vi "Check Confluence Settings.vi"(7 "Settings Path":path, 8 "Error in":errorcluster caption="Error in (no error)", 11 "Confluence Settings":T1) -> (0 "Error out":errorcluster, 3 "String":string)   [LabVIEW 2023]
uses:
  Confluence Settings.ctl
  <userlib>/_PetranWay/LabVIEW Confluence API/Source/Confluence/Confluence Connection/Confluence.lvclass
  <vilib>/DMC/VIDoc/Printers/Confluence/Confluence Printer Settings/VIDoc Settings - Confluence.lvclass
  <vilib>/DMC/VIDoc/Printers/Confluence/Confluence Printer/VIDoc Printer - Confluence.lvclass
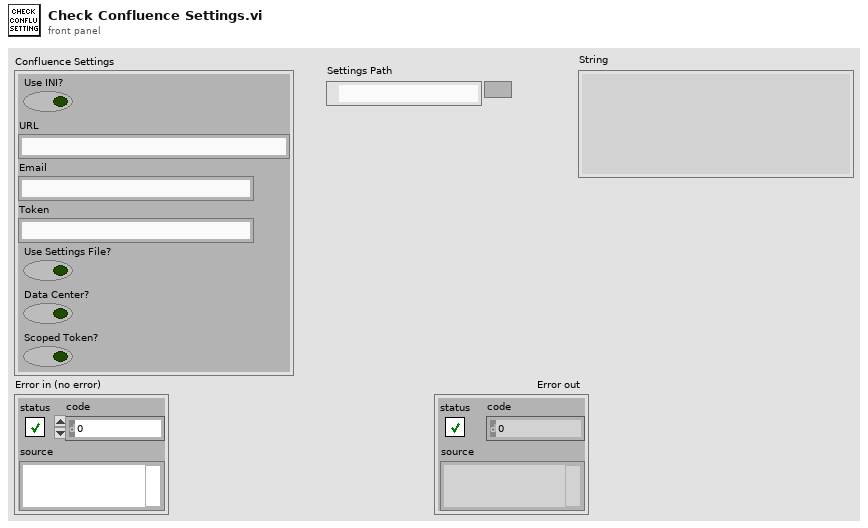
[diagram p1: front panel]
types:
  T1 = typedef "Confluence Settings.ctl" = cluster{"Use INI?":bool, "URL":string, "Email":string, "Token":string, "Use Settings File?":bool, "Data Center?":bool, "Scoped Token?":bool}
  T2 = typedef "VIDoc Printer - Confluence.lvlib/VIDoc Settings - Confluence.lvclass/Confluence Connection Settings.ctl" = cluster{"Connection Type":enum16{"Data Center", "Cloud"}, "URL":string, "Email":string}
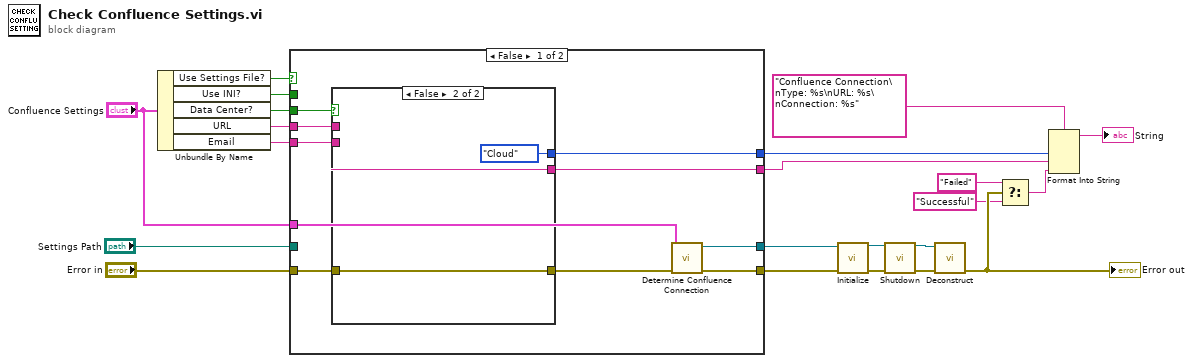
[diagram p0: block diagram]
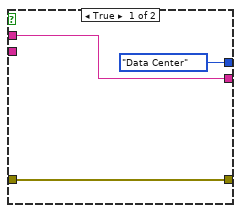
[diagram p2: hidden frame]
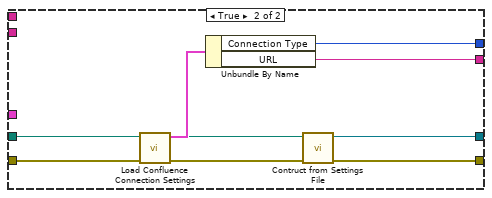
[diagram p3: hidden frame]
diagram:
  n1 = Unbundle By Name("Confluence Settings") -> ("Use Settings File?"=w22:bool, "Use INI?"=w21:bool, "Data Center?"=w20:bool, "URL"=w19:string, "Email"=w18:string)
  n2 = case shown="False" w22 {
    tunnel: [w25 w40] -> w3
    tunnel: "Error in" -> [w29 w44]
    tunnel: w21 -> [_ _]
    tunnel: w20 -> [w32 _]
    tunnel: w19 -> [w31 _]
    tunnel: w18 -> [w30 _]
    tunnel: "Settings Path" -> [_ w42]
    tunnel: [w28 w46] -> w14
    tunnel: [w27 w45] -> w13
    tunnel: [w24 w39] -> w2
    tunnel: "Confluence Settings" -> [w23 _]
    frame False {
      n3 = case shown="False" w32 {
        tunnel: w31 -> [w33 w36]
        tunnel: w30 -> [_ _]
        tunnel: w29 -> [w34 w38]
        tunnel: [w34 w38] -> w26
        tunnel: [enum16{"Data Center", "Cloud"}."Data Center" ("Connection Type") enum16{"Data Center", "Cloud"}."Cloud" ("Connection Type")] -> w28
        tunnel: [w33 w36] -> w27
        frame True {
        }
        frame False {
        }
      }
      n4 = call "Determine Confluence Connection.vi"("Error in"=w26, "Confluence Settings"=w23) -> ("Error out"=w25:errorcluster, "Confluence"=w24:refnum<class "Confluence.lvclass">)  [unwired: 8 in]
    }
    frame True {
      n5 = call <vilib>:"Load Confluence Connection Settings.vi"("Error in"=w44, "Settings Path"=w42) -> ("Error out"=w41:errorcluster, "Confluence Connection Settings"=w43:T2)  [unwired: 7 in, 1 out]
      n6 = Unbundle By Name(w43) -> ("Connection Type"=w46:enum16{"Data Center", "Cloud"}, "URL"=w45:string)
      n7 = call <vilib>:"Contruct from Settings File.vi"("Error in"=w41, "Settings Path"=w42) -> ("Error out"=w40:errorcluster, "Confluence out"=w39:refnum<class "Confluence.lvclass">)  [unwired: 8 in]
    }
  }
  n8 = call-dynamic "Initialize.vi"("Confluence in"=w2, "error in (no error)"=w3) -> ("Confluence out"=w10:refnum<class "Confluence.lvclass">, "error out"=w11:errorcluster)  [unwired: 12 in]
  n9 = call-dynamic "Shutdown.vi"("Confluence in"=w10, "error in (no error)"=w11) -> ("Confluence out"=w9:refnum<class "Confluence.lvclass">, "error out"=w8:errorcluster)  [unwired: 12 in]
  n10 = call-dynamic "Deconstruct.vi"("error in (no error)"=w8, "Confluence in"=w9) -> ("error out"=w7:errorcluster)  [unwired: 9 in]
  "Error out" <- w7
  n11 = Select(t="Failed", s=w7, f="Successful") -> (s? t:f=w4:string)
  n12 = Format Into String(format string="Confluence Connection\nType: %s\nURL: %s\nConnection: %s", w14, w13, w4) -> (resulting string=→"String":string)  [unwired: 2 in, 1 out]
